vi "DrawArmsAndPoints.vi"(11 "Array":T1(array[cluster])) -> (2 "A x B":T2=[[1.0, 0.0, 0.0, 0.0], [0.0, 6.123233995736766e-17, 1.0, 0.0], [0.0, -1.0, 6.123233995736766e-17, 0.0], [0.0, 0.0, 0.0, 1.0]] format="%#_2g", 3 "SceneObject out":refnum<vi>)   [LabVIEW 2018]
uses:
  <vilib>/Analysis/Matrix/Datatypes/RealMatrix.ctl
  <vilib>/Analysis/Matrix/NI_Matrix.lvlib
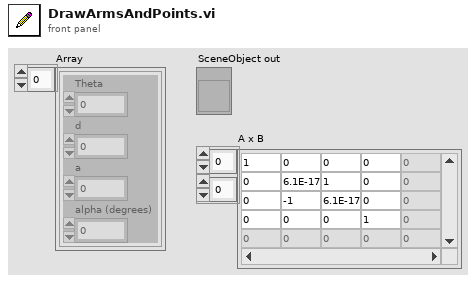
[diagram p1: front panel]
types:
  T1 = cluster{"Theta":dbl, "d":dbl, "a":dbl, "alpha (degrees)":dbl}[]
  T2 = typedef "NI_Matrix.lvlib/RealMatrix.ctl" = dbl[][]
  T3 = cluster{"Line width":sgl, "Line Color":u32, "Axes?":bool}
  T4 = cluster{"Theta (degrees)":dbl, "d":dbl, "a":dbl, "alpha (degrees)":dbl}
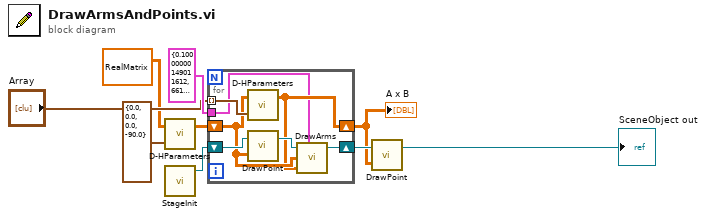
[diagram p0: block diagram]
diagram:
  n1 = call "D-HParameters.vi"("n+1"=T4 {"Theta (degrees)"=0.0, "d"=0.0, "a"=0.0, "alpha (degrees)"=-90.0}, "Start"=T2 [[1.0, 0.0, 0.0, 0.0], [0.0, 1.0, 0.0, 0.0], [0.0, 0.0, 1.0, 0.0], [0.0, 0.0, 0.0, 1.0]]) -> ("A x B"=w4:T2)  [unwired: 1 in]
  n2 = call "StageInit.vi"() -> ("Stage out"=w1:refnum<vi>)  [unwired: 4 in, 1 out]
  n3 = for {
    shift-right: [w12] -> w7
    shift-left: w4 -> [w13]
    tunnel: "Array" -> [w16] mode=indexing
    shift-right: [w10] -> w9
    shift-left: w1 -> [w15]
    tunnel: T3 {"Line width"=0.1, "Line Color"=6618880, "Axes?"=FALSE} ("Params") -> [w11]
    n4 = call "D-HParameters.vi"("n+1"=w16, "Start"=w13) -> ("A x B"=w12:T2)  [unwired: 1 in]
    n5 = call "DrawPoint.vi"("Start"=w13, "Stage in"=w15) -> ("Stage out"=w14:refnum<vi>)  [unwired: 1 in]
    n6 = call "DrawArms.vi"("Stage in"=w14, "Params"=w11, "Start"=w13, "End"=w12) -> ("Stage out"=w10:refnum<vi>)  [unwired: 2 in, 1 out]
  }
  "A x B" <- w7
  n7 = call "DrawPoint.vi"("Start"=w7, "Stage in"=w9) -> ("Stage out"=→"SceneObject out":refnum<vi>)  [unwired: 1 in]
